vi "Check Attack.vi"(11 "Maze (0: Empty, -1: Enemy. 1: Teammate":i32[](array[numeric])) -> (2 "Direction":T1, 3 "Action":T2)   [LabVIEW 2015, in "Formation.lvclass"]
uses:
  Formation.lvclass
  Type Defs/Action Enum.ctl
  Type Defs/SB Type Defs.lvlib
  Type Defs/Direction Enum.ctl
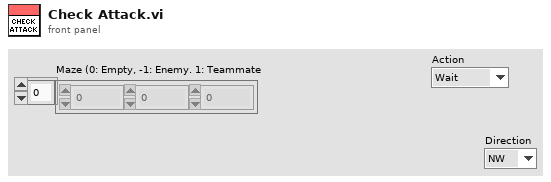
[diagram p1: front panel]
types:
  T1 = typedef "SB Type Defs.lvlib/Direction Enum.ctl" = enum16{"NW", "N", "NE", "E", "SE", "S", "SW", "W"}
  T2 = typedef "SB Type Defs.lvlib/Action Enum.ctl" = enum16{"Wait", "Move", "Attack", "Replicate"}
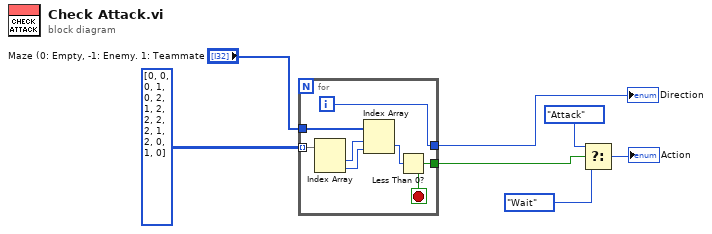
[diagram p0: block diagram]
diagram:
  n1 = for {
    tunnel: "Maze (0: Empty, -1: Enemy. 1: Teammate" -> [w14]
    tunnel: i32[][] [[0, 0], [0, 1], [0, 2], [1, 2], [2, 2], [2, 1], [2, 0], [1, 0]] -> [w13] mode=indexing
    tunnel: [w9] -> w1
    tunnel: [w8] -> w2
    i -> [w9]
    stop <- w8 stop-if-true
    n2 = Index Array(array=w13) -> (element #1=w12:i32, element #2=w11:i32)  [unwired: 2 in]
    n3 = Index Array(array=w14, index (row)=w12, index (col)=w11) -> (element=w10:i32)
    n4 = Less Than 0?(x=w10) -> (x < 0?=w8:bool)
  }
  "Direction" <- w1
  n5 = Select(t=Action_Enum."Attack" ("Action"), s=w2, f=Action_Enum."Wait") -> (s? t:f=→"Action":T2)
